vi "GDSProject_GetItemClassPath.vi"(7 "ReturnRefToClass(False)":bool, 8 "error in":errorcluster, 11 "ProjectItemRefIn":refnum<vi>) -> (0 "error out":errorcluster, 1 "LvCLassFound":bool, 2 "Path":path, 3 "ProjectItemRefOut":refnum<vi>, 4 "LvClassRef":refnum<vi>, 6 "NewRefCreated":bool)   [LabVIEW 2012]
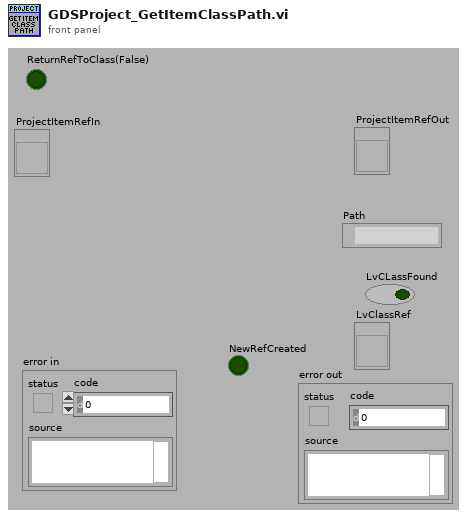
[diagram p1: front panel]
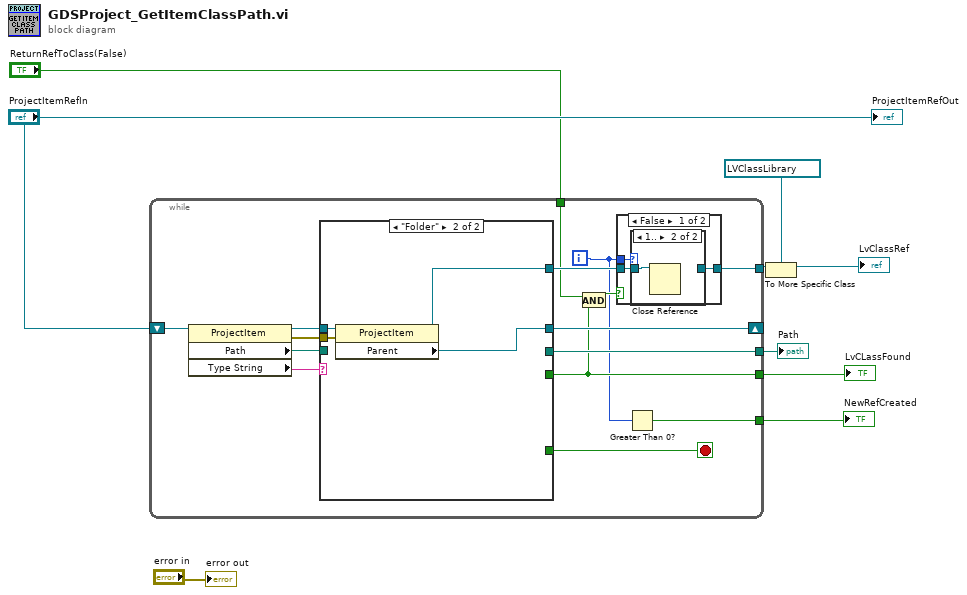
[diagram p0: block diagram]
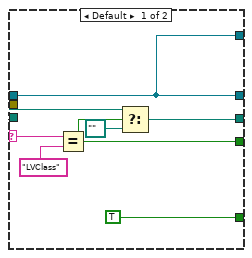
[diagram p4: hidden frame]
diagram:
  n1 = while {
    shift-right: [w24] -> _
    shift-left: "ProjectItemRefIn" -> [w22]
    tunnel: [w13] -> w8
    tunnel: [w16] -> w6
    tunnel: [w15] -> w5
    tunnel: "ReturnRefToClass(False)" -> [w12]
    tunnel: [w10] -> w1
    i -> [w11]
    stop <- w23 stop-if-true
    n2 = property class="ProjectItem"(reference=w22) -> (reference out=w21:refnum<vi>, error out=w20:errorcluster, "Path"=w17:path, "Type String"=w19:string)  [unwired: 1 in]
    n3 = case shown="\"Folder\"" w19 {
      selector: w19 -> [w35 _]
      tunnel: [w37 w40] -> w24
      tunnel: [TRUE _] -> w23
      tunnel: w21 -> [w37 w42]
      tunnel: w20 -> [_ w41]
      tunnel: [w37 w39] -> w18
      tunnel: [w34 _] -> w13
      tunnel: w17 -> [w33 _]
      tunnel: [w32 _] -> w16
      frame Default {
        n4 = Equal?(x=w35, y="LVClass" ("x")) -> (x = y?=w34:bool)
        n5 = Select(t=w33, s=w34, f=path "") -> (s? t:f=w32:path)
      }
      frame "Folder" {
        n6 = property class="ProjectItem"(reference=w42, error in=w41) -> (reference out=w39:refnum<vi>, "Parent"=w40:refnum<vi>)  [unwired: 1 out]
      }
    }
    n7 = And(x=w12, y=w13) -> (x .and. y?=w14:bool)
    n8 = case shown="False" w14 {
      tunnel: w11 -> [w27 _]
      tunnel: w18 -> [w26 w30]
      tunnel: [w25 w30] -> w15
      frame False {
        n9 = case shown="1.." w27 {
          tunnel: w26 -> [w28 w29]
          tunnel: [w28 _] -> w25
          frame 0, Default {
          }
          frame 1.. {
            n10 = Close Reference(reference=w29) -> ()  [unwired: 1 in, 1 out]
          }
        }
      }
      frame True {
      }
    }
    n11 = Greater Than 0?(x=w11) -> (x > 0?=w10:bool)
  }
  "LvCLassFound" <- w8
  "Path" <- w6
  "NewRefCreated" <- w1
  n12 = To More Specific Class(target class=refnum<vi> refnum ("LvClassRef"), reference=w5) -> (specific class reference=→"LvClassRef":refnum<vi>)  [unwired: 1 in, 1 out]
  "ProjectItemRefOut" <- "ProjectItemRefIn"
  "error out" <- "error in"
